vi "target - multi rate - variables.vi"   [LabVIEW 2010]
uses:
  <vilib>/Platform/TimedLoop/XDataNode/XDataNode.xnode
  <vilib>/Platform/TimedLoop/XDataNode/timing_clust.ctl
  <vilib>/Platform/TimedLoop/XDataNode/nitl_modes.ctl
  <vilib>/Platform/TimedLoop/XDataNode/wakeup.ctl
  <vilib>/Platform/TimedLoop/XDataNode/XDNodeRunTimeDep.lvlib
panel:
  # "The Network Variable Engine and Variable Client Support must be installed on the RT target\nfor this application to function properly. If the Network Variable Engine is not supported on\nthe target (e.g.  FP-2000 with <32MB of RAM), open the project and move the variable library\nto My Computer in the project. Doing this will deploy the variables to localhost but\nwill still require that Variable Client Support be installed on the RT target."
types:
  T1 = typedef "XDNodeRunTimeDep.lvlib/timing_clust.ctl" = cluster{"Expected End [f-1]":u64, "Actual End [f-1]":u64, "Finished Late? [f-1]":bool, "Expected End [i-1]":u64, "Actual End [i-1]":u64, "Finished Late? [i-1]":bool, "Expected Start [i]":u64, "Actual Start [i]":u64, "Expected Start [f]":u64, "Actual Start [f]":u64, "Source Name":string, "Structure Name":string, "Period":i64, "Deadline":i64, "Offset":i64, "Start":i64, "Priority":i32, "Timeout":i32, "Mode":T2, "Wakeup Reason":T3, "Error":errorcluster, "Source Type":string, "Secondary Source Type":string, "Global End Time":u64, "Global Start Time":u64, "Frame Duration":u64, "Iteration Duration":u64, "Assigned CPU":i32, "I/O Scan Engine Mode":u32}
  T2 = typedef "XDNodeRunTimeDep.lvlib/nitl_modes.ctl" = enum32{"No Change", "Process missed periods, maintain original phase", "Discard missed periods, maintain original phase", "Process missed periods, ignore original phase", "Discard missed periods, ignore original phase"}
  T3 = typedef "XDNodeRunTimeDep.lvlib/wakeup.ctl" = enum32{"Normal", "Aborted", "Asynchronous wakeup", "Timing source error", "Timed loop error", "Timeout"}
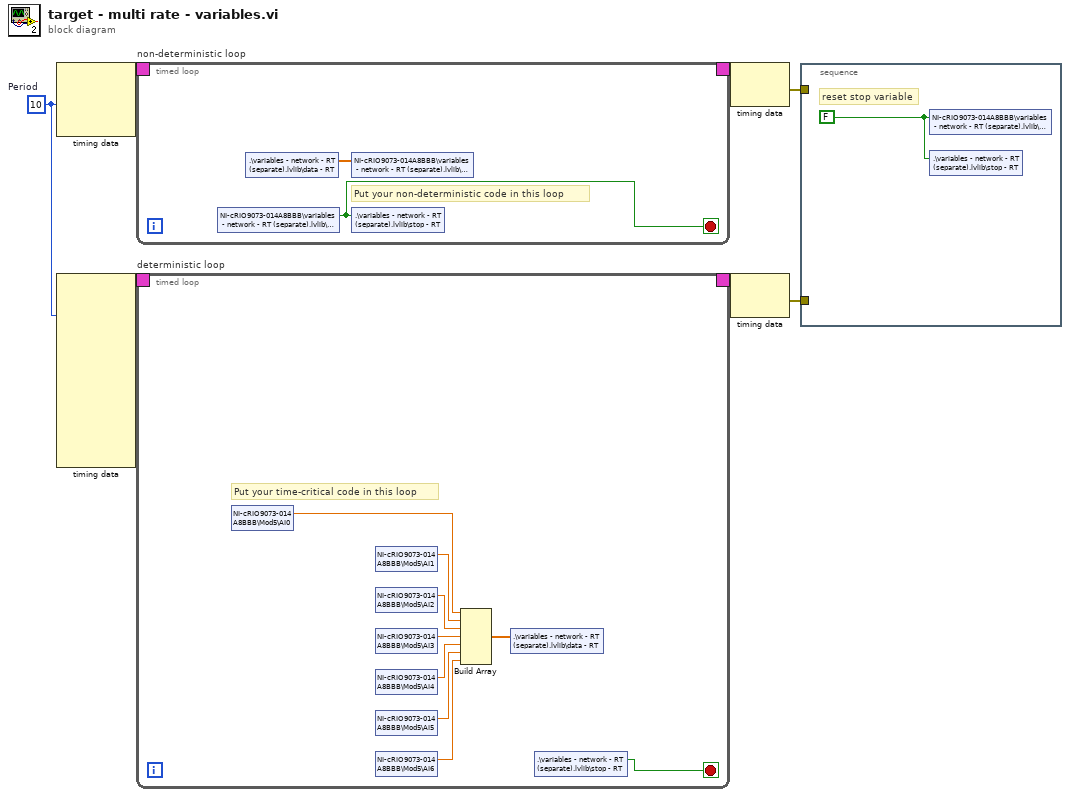
[diagram p0: block diagram]
diagram:
  w3 = i64 10  # Period
  n1 = node-c288 ("Input Node")(w3) -> (w5:T1)  [unwired: 2 in]
  n2 = node-c288 ("Input Node")(w3) -> (w7:T1)  [unwired: 9 in]
  n3 = timed-loop "non-deterministic loop" {
    timing: w5 -> [_]
    timing-out: [_] -> w4
    stop <- w8 stop-if-true
    # "Put your non-deterministic code in this loop"
    n4 = shared-variable "NI-cRIO9073-014A8BBB\\variables - network - RT (separate).lvlib\\stop - network"() -> (w8:bool)  [unwired: 1 in, 1 out]
    n5 = shared-variable ".\\variables - network - RT (separate).lvlib\\data - RT"() -> (w9:dbl[])  [unwired: 1 in, 1 out]
    n6 = shared-variable "NI-cRIO9073-014A8BBB\\variables - network - RT (separate).lvlib\\data - network"(w9) -> ()  [unwired: 1 in, 1 out]
    n7 = shared-variable ".\\variables - network - RT (separate).lvlib\\stop - RT"(w8) -> ()  [unwired: 1 in, 1 out]
  }
  n8 = timed-loop "deterministic loop" {
    timing: w7 -> [_]
    timing-out: [_] -> w6
    stop <- w20 stop-if-true
    # "Put your time-critical code in this loop"
    n9 = shared-variable "NI-cRIO9073-014A8BBB\\Mod5\\AI0"() -> (w19:dbl)  [unwired: 1 in, 1 out]
    n10 = shared-variable "NI-cRIO9073-014A8BBB\\Mod5\\AI1"() -> (w18:dbl)  [unwired: 1 in, 1 out]
    n11 = shared-variable "NI-cRIO9073-014A8BBB\\Mod5\\AI2"() -> (w17:dbl)  [unwired: 1 in, 1 out]
    n12 = shared-variable "NI-cRIO9073-014A8BBB\\Mod5\\AI3"() -> (w16:dbl)  [unwired: 1 in, 1 out]
    n13 = shared-variable "NI-cRIO9073-014A8BBB\\Mod5\\AI4"() -> (w15:dbl)  [unwired: 1 in, 1 out]
    n14 = shared-variable "NI-cRIO9073-014A8BBB\\Mod5\\AI5"() -> (w14:dbl)  [unwired: 1 in, 1 out]
    n15 = shared-variable "NI-cRIO9073-014A8BBB\\Mod5\\AI6"() -> (w13:dbl)  [unwired: 1 in, 1 out]
    n16 = Build Array(w19, w18, w17, w16, w15, w14, w13) -> (w12:dbl[])
    n17 = shared-variable ".\\variables - network - RT (separate).lvlib\\data - RT"(w12) -> ()  [unwired: 1 in, 1 out]
    n18 = shared-variable ".\\variables - network - RT (separate).lvlib\\stop - RT"() -> (w20:bool)  [unwired: 1 in, 1 out]
  }
  n19 = node-c288 ("Output Node")(w4) -> (w1:errorcluster)
  n20 = node-c288 ("Output Node")(w6) -> (w2:errorcluster)
  n21 = stacked-sequence {
    tunnel: w2 -> [_]
    tunnel: w1 -> [_]
    frame #0 {
      w23 = FALSE
      # "reset stop variable"
      n22 = shared-variable "NI-cRIO9073-014A8BBB\\variables - network - RT (separate).lvlib\\stop - network"(w23) -> ()  [unwired: 1 in, 1 out]
      n23 = shared-variable ".\\variables - network - RT (separate).lvlib\\stop - RT"(w23) -> ()  [unwired: 1 in, 1 out]
    }
  }
